vi "ILABW_AppStatus.vi"() -> (3 "output":string)   [LabVIEW 2012]
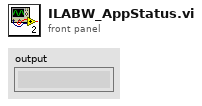
[diagram p1: front panel]
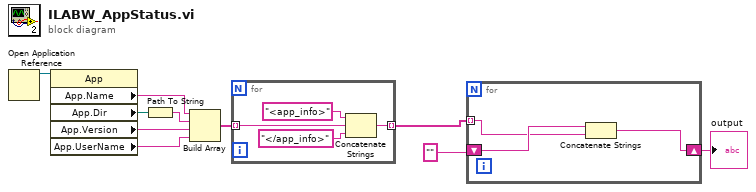
[diagram p0: block diagram]
diagram:
  n1 = Open Application Reference() -> (3:w10:refnum<vi>)  [unwired: 4 in, 1 out]
  n2 = property class="App"(reference=w10) -> ("App.Name"=w8:string, "App.Dir"=w9:path, "App.Version"=w6:string, "App.UserName"=w5:string)  [unwired: 1 in, 2 out]
  n3 = Path To String(path=w9) -> (string=w7:string)
  n4 = Build Array(w8, w7, w6, w5) -> (w4:string[])
  n5 = for {
    tunnel: w4 -> [w14] mode=indexing
    tunnel: [w13] -> w3 mode=indexing
    n6 = Concatenate Strings("<app_info>" ("string"), w14, "</app_info>" ("string")) -> (w13:string)
  }
  n7 = for {
    tunnel: w3 -> [w16] mode=indexing
    shift-right: [w15] -> w1
    shift-left: "" -> [w17]
    n8 = Concatenate Strings(w17, w16) -> (w15:string)
  }
  "output" <- w1
